vi "Package External Actuator Data.vi"(9 "External Actuator Commands In":dbl[](array[numeric]), 11 "External Actuator Readings In":dbl[](array[numeric])) -> (1 "Right External Actuator Data Out":T1, 3 "Left External Actuator Data Out":T1)   [LabVIEW 2009]
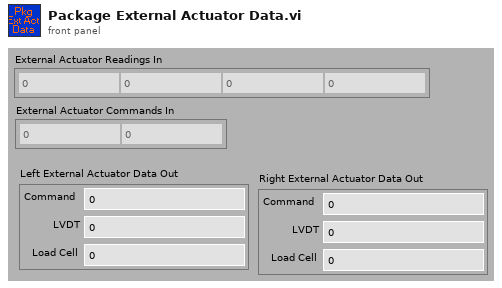
[diagram p1: front panel]
types:
  T1 = cluster{"Command":dbl, "LVDT":dbl, "Load Cell":dbl}
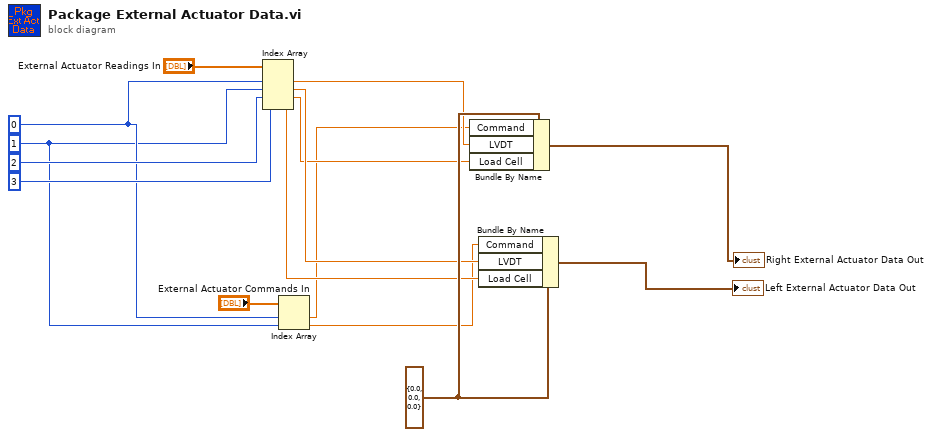
[diagram p0: block diagram]
diagram:
  w5 = 1 ("index")
  w6 = 0 ("index")
  w12 = T1 {"Command"=0.0, "LVDT"=0.0, "Load Cell"=0.0} ("Right External Actuator Data Out")
  n1 = Index Array(array="External Actuator Readings In", index #1=w6, index #2=w5, index #3=2 ("index"), index #4=3 ("index")) -> (element #1=w11:dbl, element #2=w10:dbl, element #3=w8:dbl, element #4=w9:dbl)
  n2 = Index Array(array="External Actuator Commands In", index #1=w6, index #2=w5) -> (element #1=w4:dbl, element #2=w3:dbl)
  n3 = Bundle By Name(cluster=w12, "Command"=w4, "LVDT"=w11, "Load Cell"=w8) -> (→"Right External Actuator Data Out":T1)
  n4 = Bundle By Name(cluster=w12, "Command"=w3, "LVDT"=w10, "Load Cell"=w9) -> (→"Left External Actuator Data Out":T1)
